vi "r_to_t.vi"(1 "T equation":string="197.4556-51.4464*log(x)", 3 "Resistance":dbl) -> (0 "Temperature":dbl)   [LabVIEW 2010]
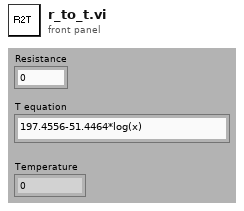
[diagram p1: front panel]
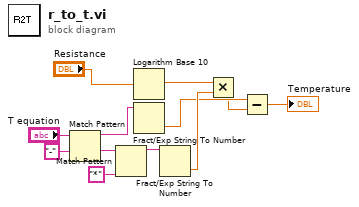
[diagram p0: block diagram]
diagram:
  n1 = Match Pattern(string="T equation", regular expression="-") -> (before substring=w8:string, after substring=w10:string)  [unwired: 1 in, 2 out]
  n2 = Match Pattern(string=w10, regular expression="*") -> (before substring=w7:string)  [unwired: 1 in, 3 out]
  n3 = Logarithm Base 10(1:"Resistance") -> (0:w6:dbl)
  n4 = Fract/Exp String To Number(string=w8) -> (number=w4:dbl)  [unwired: 3 in, 1 out]
  n5 = Fract/Exp String To Number(string=w7) -> (number=w5:dbl)  [unwired: 3 in, 1 out]
  n6 = Multiply(x=w6, y=w5) -> (x*y=w3:dbl)
  n7 = Subtract(x=w4, y=w3) -> (x-y=→"Temperature":dbl)
